vi "Create MF4 File_Ch.vi"(7 "DLL path":path, 8 "Error In":errorcluster, 11 "input cluster":T1) -> (0 "Error Out":errorcluster, 1 "Stream Reference out":i64, 2 "Channels Count":i32, 3 "MDF4 File Reference out":i64)   [LabVIEW 2019, in "MD4Logger Engine.lvlib"]
uses:
  MD4Logger Engine.lvlib
  Shared/Compiled.Settings.ctl
  Shared/MD4Logger Shared.lvlib
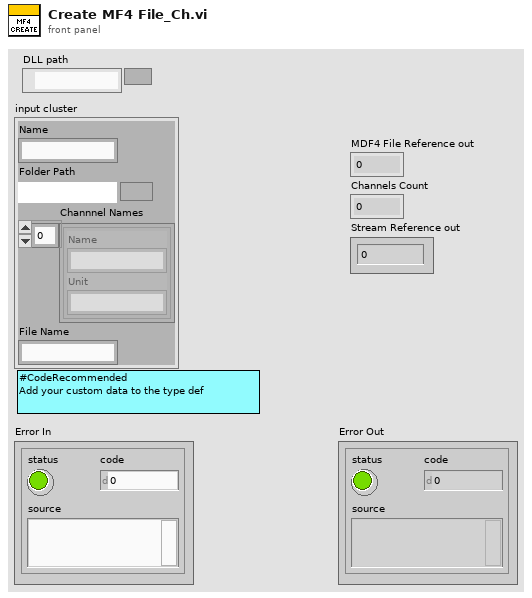
[diagram p1: front panel]
types:
  T1 = typedef "MD4Logger Shared.lvlib/Compiled.Settings.ctl" = cluster{"Name":string, "Folder Path":path, "Channnel Names":cluster{"Name":string, "Unit":string}[], "File Name":string}
  T2 = cluster{"History":string, "ID":string, "Vendor":string, "Version":string}
  T3 = cluster{"Comment":string, "Time Source":string, "Author":string, "Department":string, "Project":string, "Subject":string}
  T4 = typedef "LVDateTimeRec.ctl" = cluster{"fractional second":dbl, "second":i32, "minute":i32, "hour":i32, "day of month":i32, "month":i32, "year":i32, "day of week":i32, "day of year":i32, "DST":i32}
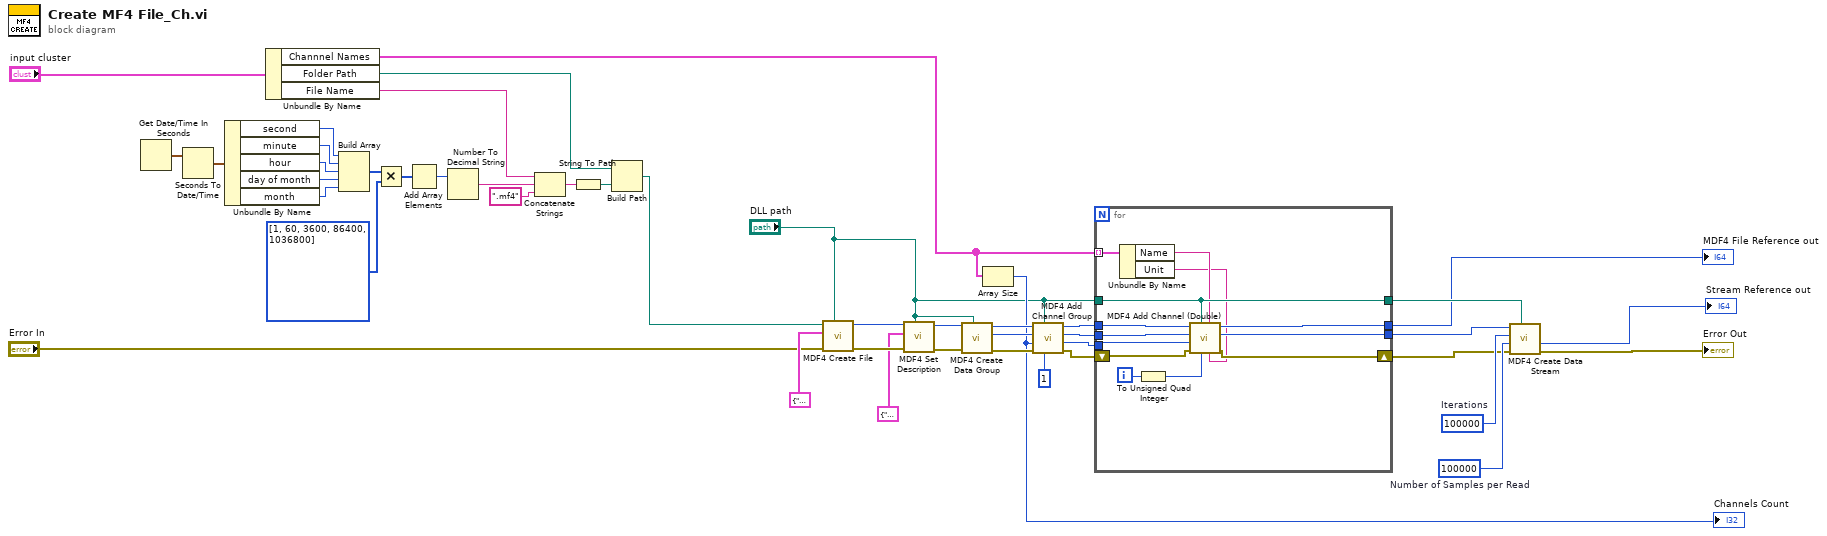
[diagram p0: block diagram]
diagram:
  w12 = u32 100000  # Iterations
  w13 = u32 100000  # Number of Samples per Read
  n1 = Get Date/Time In Seconds() -> (seconds since 1Jan1904=w38:timestamp)
  n2 = Seconds To Date/Time(time stamp (now)=w38) -> (date time rec=w37:T4)  [unwired: 1 in]
  n3 = Unbundle By Name(w37) -> ("second"=w36:i32, "minute"=w35:i32, "hour"=w34:i32, "day of month"=w33:i32, "month"=w32:i32)
  n4 = Unbundle By Name("input cluster") -> ("Channnel Names"=w14:cluster{"Name":string, "Unit":string}[], "Folder Path"=w15:path, "File Name"=w7:string)
  n5 = Build Array(w36, w35, w34, w33, w32) -> (w31:i32[])
  n6 = Multiply(x=w31, y=i32[] [1, 60, 3600, 86400, 1036800]) -> (x*y=w29:i32[])
  n7 = Add Array Elements(numeric array=w29) -> (sum=w28:i32)
  n8 = Number To Decimal String(number=w28) -> (decimal integer string=w27:string)  [unwired: 1 in]
  n9 = Concatenate Strings(w7, w27, ".mf4" ("string")) -> (w25:string)
  n10 = String To Path(string=w25) -> (path=w24:path)
  n11 = Build Path(base path=w15, name or relative path=w24) -> (appended path=w39:path)
  n12 = call "MDF4 Create File.vi"("path in"="DLL path", "Error In"="Error In", "History"=T2 {"History"="my History", "ID"="LabVIEW Logger", "Vendor"="National Instruments", "Version"="1.0"}, "MDF4 File Path"=w39) -> ("Error Out"=w42:errorcluster, "MDF4 File Reference out"=w43:i64)  [unwired: 5 in]
  n13 = call "MDF4 Set Description.vi"("path in"="DLL path", "Error In"=w42, "Comment"=T3 {"Comment"="my comment", "Time Source"="Local PC Reference Time", "Author"="Author", "Department"="Department", "Project"="Project", "Subject"="Subject"}, "MDF4 File Reference in"=w43) -> ("Error Out"=w45:errorcluster, "MDF4 File Reference out"=w44:i64)  [unwired: 6 in]
  n14 = call "MDF4 Create Data Group.vi"("path in"="DLL path", "Error In"=w45, "MDF4 File Reference in"=w44) -> ("Error Out"=w23:errorcluster, "Data Group Reference out"=w22:i64, "MDF4 File Reference out"=w21:i64)  [unwired: 6 in]
  n15 = Array Size(array=w14) -> (size(s)=w8:i32)
  "Channels Count" <- w8
  n16 = call "MDF4 Add Channel Group.vi"("Record ID"=u64 1, "path in"="DLL path", "Error In"=w23, "chan_count"=w8, "Data Group Reference in"=w22, "MDF4 File Reference in"=w21) -> ("Error Out"=w20:errorcluster, "Channel Group Reference out"=w17:i64, "Data Group Reference out"=w18:i64, "MDF4 File Reference out"=w19:i64)  [unwired: 2 in]
  n17 = for {
    tunnel: [w51] -> w4
    shift-right: [w56] -> w11
    shift-left: w20 -> [w55]
    tunnel: w19 -> [w47]
    tunnel: w18 -> [w48]
    tunnel: w17 -> [w49]
    tunnel: w14 -> [w57] mode=indexing
    tunnel: "DLL path" -> [w53]
    tunnel: [w53] -> w9
    tunnel: [w50] -> w10
    i -> [w58]
    n18 = Unbundle By Name(w57) -> ("Name"=w52:string, "Unit"=w46:string)
    n19 = To Unsigned Quad Integer(1:w58) -> (0:w54:u64)
    n20 = call "MDF4 Add Channel (Double).vi"("Channel Unit"=w46, "Channel Name"=w52, "chan_index"=w54, "path in"=w53, "Error In"=w55, "Channel Group Reference in"=w49, "Data Group Reference in"=w48, "MDF4 File Reference in"=w47) -> ("Error Out"=w56:errorcluster, "Data Group Reference out"=w50:i64, "MDF4 File Reference out"=w51:i64)  [unwired: 1 in]
  }
  "MDF4 File Reference out" <- w4
  n21 = call "MDF4 Create Data Stream.vi"("path in"=w9, "Error In"=w11, "Number of Samples per Read"=w13, "Iterations"=w12, "Data Group Reference in"=w10) -> ("Error Out"=→"Error Out":errorcluster, "Stream Reference out"=→"Stream Reference out":i64)  [unwired: 4 in, 1 out]
